vi "Cooler OFF.vi"(8 "error in (no error)":errorcluster, 11 "Cooler in":refnum<class "Cooler.lvclass">) -> (0 "error out":errorcluster, 3 "Cooler out":refnum<class "Cooler.lvclass">)   [LabVIEW 2018, in "Cooler.lvclass"]
uses:
  Cooler.lvclass
  C:/Users/observer/Desktop/SPARC4_ACS/Simulated_Cooler/Simulated_Cooler.lvclass
  Simulated_Cooler/Simulated_Cooler.lvclass/Simulated_Cooler.ctl
  Simulated_Cooler/Simulated_Cooler.lvclass
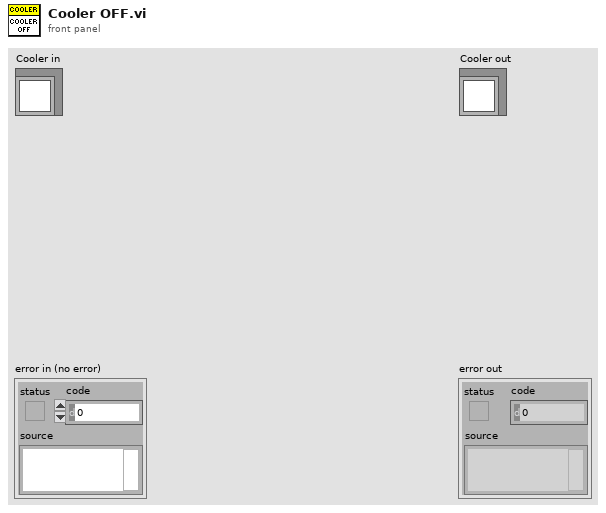
[diagram p1: front panel]
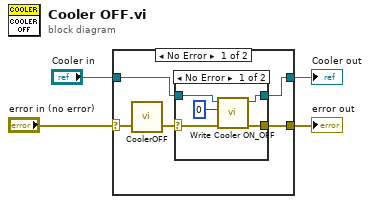
[diagram p0: block diagram]
diagram:
  n1 = case shown="No Error" "error in (no error)" {
    selector: "error in (no error)" -> [w9 w18]
    tunnel: [w7 w18] -> w3
    tunnel: [w5 w17] -> w1
    tunnel: "Cooler in" -> [w6 w17]
    frame No Error {
      n2 = call <userlib>:"CoolerOFF.vi"("error in (no error)"=w9) -> ("error out"=w8:errorcluster)  [unwired: 1 in, 1 out]
      n3 = case shown="No Error" w8 {
        selector: w8 -> [w14 w15]
        tunnel: [w13 w15] -> w7
        tunnel: w6 -> [w11 w16]
        tunnel: [w12 w16] -> w5
        frame No Error {
          n4 = call "Write Cooler ON_OFF.vi"("error in (no error)"=w14, "Cooler ON/OFF"=u8 0, "Cooler in"=w11) -> ("error out"=w13:errorcluster, "Cooler out"=w12:refnum<class "Cooler.lvclass">)  [unwired: 7 in]
        }
        frame Error {
        }
      }
    }
    frame Error {
    }
  }
  "error out" <- w3
  "Cooler out" <- w1
